vi "UART Read.vi"(8 "Error In":errorcluster, 9 "Num Bytes":u8, 10 "UART Channel":u8, 11 "LINX Device Config":T1) -> (0 "Error Out":errorcluster, 2 "Data":u8[](array[numeric]), 3 "LINX Device Config":T1)   [LabVIEW 2013, in "LVH-LINX.lvlib" / "Device.lvlib"]
doc: "Read the specified number of bytes from the specified UART channel's receive buffer."
uses:
  <vilib>/LabVIEW Hacker/LINX/Private/Device/Device.lvlib
  <vilib>/LabVIEW Hacker/LINX/Private/Device/Type Defs/LINX Device Config.ctl
  <vilib>/LabVIEW Hacker/LINX/Private/Type Defs/Interface.ctl
  <vilib>/LabVIEW Hacker/LINX/Private/Device/Type Defs/TCP Config.ctl
  <vilib>/LabVIEW Hacker/LINX/Private/Type Defs/Device Family.ctl
  <vilib>/LabVIEW Hacker/LINX/Private/Type Defs/Error Type.ctl
  <vilib>/LabVIEW Hacker/LINX/LVH-LINX.lvlib
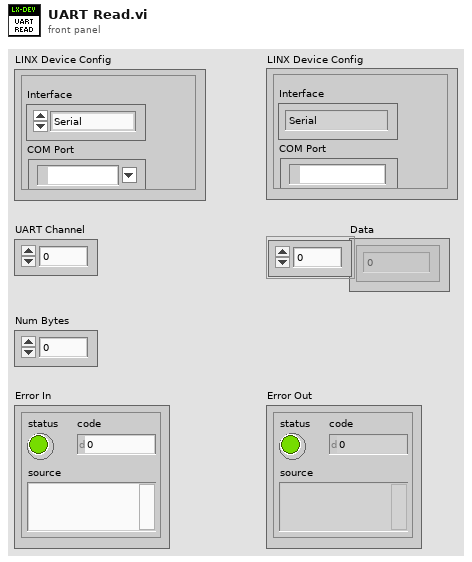
[diagram p1: front panel]
types:
  T1 = typedef "LVH-LINX.lvlib/Device.lvlib/LINX Device Config.ctl" = cluster{"Interface":T2, "COM Port":refnum<visa-resource-name>, "TCP Configuration":T3, "Device Family":T4, "Device ID":u8, "Device Name":string, "TCP Ref":refnum<k5>}
  T2 = typedef "LVH-LINX.lvlib/Interface.ctl" = enum16{"Serial", "TCP"}
  T3 = typedef "LVH-LINX.lvlib/Device.lvlib/TCP Config.ctl" = cluster{"IP Address":string, "Port":u16}
  T4 = typedef "LVH-LINX.lvlib/Device Family.ctl" = enum8{"National Instruments", "Digilent", "Arduino"}
  T5 = typedef "LVH-LINX.lvlib/Error Type.ctl" = enum16{"Unknown", "Timeout", "Corrupt Return Packet", "Unable To Connect", "Command Not Supported", "Channel DNE", "Invalid COM Config"}
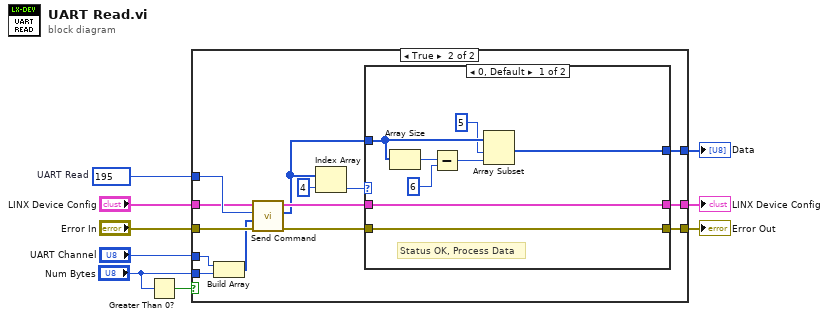
[diagram p0: block diagram]
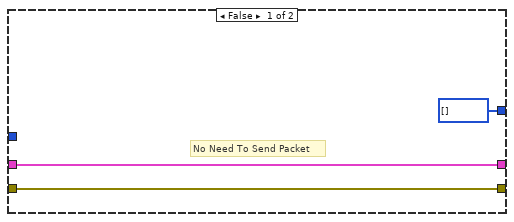
[diagram p2: hidden frame]
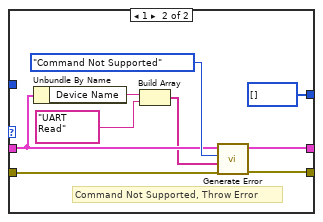
[diagram p3: hidden frame]
diagram:
  w8 = u16 195  # UART Read
  n1 = Greater Than 0?(x="Num Bytes") -> (x > 0?=w1:bool)
  n2 = case shown="True" w1 {
    tunnel: "Error In" -> [w12 w26]
    tunnel: w8 -> [_ w25]
    tunnel: "LINX Device Config" -> [w11 w24]
    tunnel: [w11 w21] -> w6
    tunnel: [w12 w19] -> w5
    tunnel: "UART Channel" -> [_ w17]
    tunnel: "Num Bytes" -> [_ w15]
    tunnel: [u8[] [] w13] -> w3
    frame False {
      # "No Need To Send Packet"
    }
    frame True {
      n3 = Build Array(w17, w15) -> (w16:u8[])
      n4 = call <vilib>:"Send Command.vi"("Error In"=w26, "ARGS"=w16, "CMD"=w25, "LINX Device Config"=w24) -> ("Error Out"=w18:errorcluster, "Response"=w14:u8[], "LINX Device Config"=w20:T1)  [unwired: 4 in, 1 out]
      n5 = Index Array(array=w14, index=4) -> (element=w22:u8)
      n6 = case shown="0, Default" w22 {
        tunnel: [w34 w41] -> w21
        tunnel: w20 -> [w34 w37]
        tunnel: [w33 w42] -> w19
        tunnel: w18 -> [w33 w43]
        tunnel: w14 -> [w29 _]
        tunnel: [w27 u8[] []] -> w13
        frame 0, Default {
          # "Status OK, Process Data"
          n7 = Array Size(array=w29) -> (size(s)=w32:i32)
          n8 = Subtract(x=w32, y=6) -> (x-y=w30:i32)
          n9 = Array Subset(array=w29, index=5, length=w30) -> (w27:u8[])
        }
        frame 1 {
          # "Command Not Supported, Throw Error"
          n10 = Unbundle By Name(w37) -> ("Device Name"=w39:string)
          n11 = Build Array(w39, "UART Read") -> (w36:string[])
          n12 = call <vilib>:"Generate Error.vi"("Error In"=w43, "Arguments"=w36, "Error Type"=Error_Type."Command Not Supported", "LINX Device Config"=w37) -> ("Error Out"=w42:errorcluster, "LINX Device Config"=w41:T1)  [unwired: 6 in]
        }
      }
    }
  }
  "Error Out" <- w5
  "LINX Device Config" <- w6
  "Data" <- w3
